vi "get superNode.vi"(8 "error in (no error)":errorcluster, 11 "xceNode in":refnum<class "xceNode.lvclass">) -> (0 "error out":errorcluster, 2 "superNode*":refnum<data-value>, 3 "xceNode out":refnum<class "xceNode.lvclass">)   [LabVIEW 2013, in "xceNode.lvclass"]
doc: "Gets superNode. superNode is a data value reference to an xceNode that resides above this node in the tree data structure."
uses:
  xceNode.lvclass
  xceTreeObj/xceTreeObj.lvclass
  xceNode.lvclass/xceNode.ctl
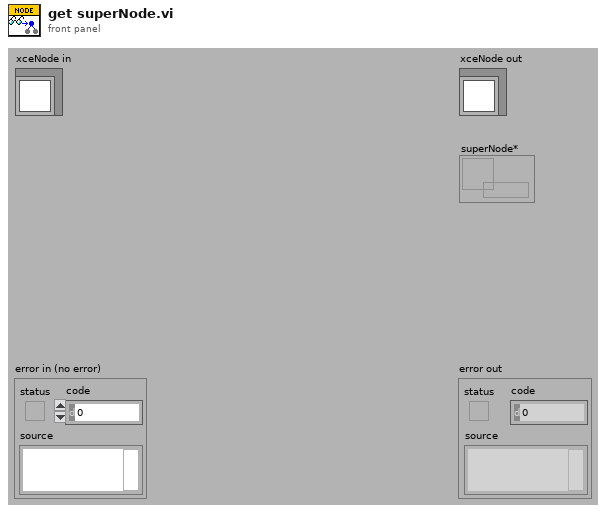
[diagram p1: front panel]
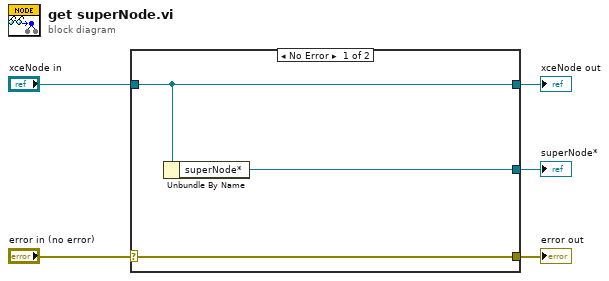
[diagram p0: block diagram]
diagram:
  n1 = case shown="No Error" "error in (no error)" {
    selector: "error in (no error)" -> [w8 w9]
    tunnel: [w8 w9] -> w4
    tunnel: [w7 w10] -> w2
    tunnel: "xceNode in" -> [w7 w10]
    tunnel: [w6 _] -> w1
    frame No Error {
      n2 = Unbundle By Name(w7) -> ("superNode*"=w6:refnum<data-value>)
    }
    frame Error {
    }
  }
  "error out" <- w4
  "xceNode out" <- w2
  "superNode*" <- w1
